vi "PCO_RecorderGetVersion.vi"(8 "error in (no error)":errorcluster {"code" format="%x"}) -> (0 "error out":errorcluster {"code" format="%x"}, 1 "iPatch":i32, 2 "iMinor":i32, 3 "iMajor":i32, 5 "iBuild":i32)   [LabVIEW 2020, in "Recorder.lvlib"]
doc: "void WINAPI PCO_RecorderGetVersion(int* iMajor, int* iMinor, int* iPatch, int* iBuild);"
uses:
  Recorder.lvlib
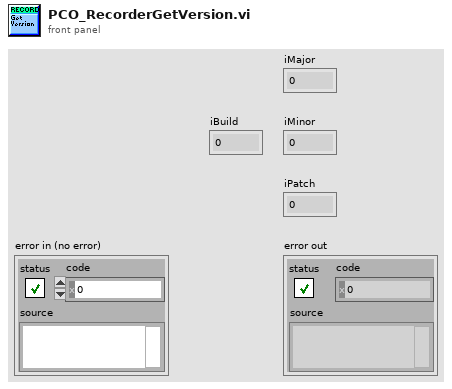
[diagram p1: front panel]
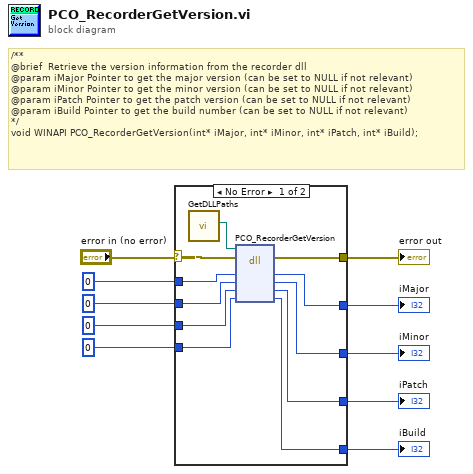
[diagram p0: block diagram]
diagram:
  # "/**\n@brief  Retrieve the version information from the recorder dll\n@param iMajor Pointer to get the major version (can be set to NULL if not relevant)\n@param iMinor Pointer to get the minor version (can be set to NULL if not relevant)\n@param iPatch Pointer to get the patch version (can be set to NULL if not relevant)\n@param iBuild Pointer to get the build number (can be set to NULL if not relevant)\n*/\nvoid WINAPI PCO_RecorderGetVersion(int* iMajor, int* iMinor, int* iPatch, int* iBuild);"
  n1 = case shown="No Error" "error in (no error)" {
    selector: "error in (no error)" -> [w12 w26]
    tunnel: 0 ("iMajor") -> [w21 w25]
    tunnel: [w20 w25] -> w9
    tunnel: 0 ("iMinor") -> [w19 w24]
    tunnel: [w18 w24] -> w7
    tunnel: 0 ("iPatch") -> [w17 w23]
    tunnel: [w16 w23] -> w5
    tunnel: 0 ("iBuild") -> [w15 w22]
    tunnel: [w14 w22] -> w3
    tunnel: [w13 w26] -> w2
    frame No Error {
      n2 = call "GetDLLPaths.vi"() -> ("PCO_Recorder_Path"=w11:path)  [unwired: 9 in, 2 out]
      n3 = dll-call lib="?" fn="PCO_RecorderGetVersion"(path in=w11, error in=w12, "iMajor"=w21, "iMinor"=w19, "iPatch"=w17, "iBuild"=w15) -> (error out=w13:errorcluster, "iMajor"=w20:i32, "iMinor"=w18:i32, "iPatch"=w16:i32, "iBuild"=w14:i32)  [unwired: 2 in, 1 out]
    }
    frame Error {
    }
  }
  "iMajor" <- w9
  "iMinor" <- w7
  "iPatch" <- w5
  "iBuild" <- w3
  "error out" <- w2
